vi "LOERN_OnOperate.vi"(0 "XRef":T8, 1 "Point":T6, 2 "State In":T1={"Inputs"=1, "SelectedIndex"=1, "ClassInfo"=[]}) -> (14 "Reply":T4, 15 "Fatal Error Out":T3, 16 "State Out":T1={"Inputs"=1, "SelectedIndex"=1, "ClassInfo"=[]})   [LabVIEW 2016, in "LV Object Event Registration Node.xnode"]
uses:
  LV Object Event Registration Node.xnode
  <vilib>/XNodeSupport/XNodeXNodeRef.ctl
  <vilib>/XNodeSupport/XNodePoint.ctl
  <vilib>/XNodeSupport/XNodeInt.ctl
  LOERN_State.ctl
  LOERN_ClassInfo.ctl
  <vilib>/XNodeSupport/XNodeStringArray.ctl
  <vilib>/XNodeSupport/XNodeString.ctl
  <vilib>/XNodeSupport/XNodeErrorCluster.ctl
  <vilib>/XNodeSupport/NI_XNodeSupport.lvlib
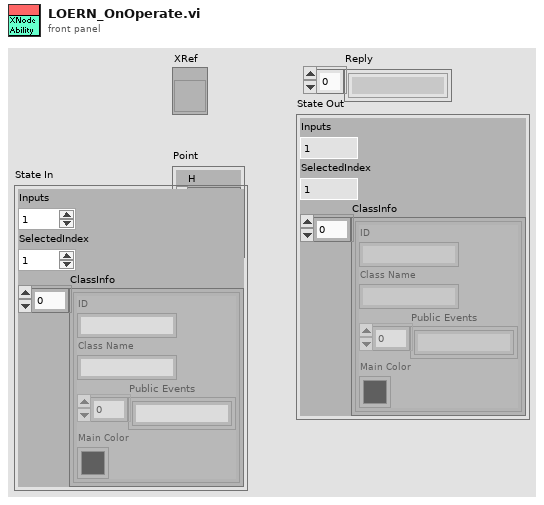
[diagram p1: front panel]
types:
  T1 = typedef "LV Object Event Registration Node.xnode/LOERN_State.ctl" = cluster{"Inputs":u16, "SelectedIndex":i16, "ClassInfo":T2[]}
  T2 = typedef "LV Object Event Registration Node.xnode/LOERN_ClassInfo.ctl" = cluster{"ID":string, "Class Name":string, "Public Events":string[], "Main Color":u32}
  T3 = typedef "NI_XNodeSupport.lvlib/XNodeErrorCluster.ctl" = errorcluster
  T4 = typedef "NI_XNodeSupport.lvlib/XNodeStringArray.ctl" = T5[]
  T5 = typedef "NI_XNodeSupport.lvlib/XNodeString.ctl" = string
  T6 = typedef "NI_XNodeSupport.lvlib/XNodePoint.ctl" = cluster{"H":T7, "V":T7}
  T7 = typedef "NI_XNodeSupport.lvlib/XNodeInt.ctl" = i32
  T8 = typedef "NI_XNodeSupport.lvlib/XNodeXNodeRef.ctl" = refnum<vi>
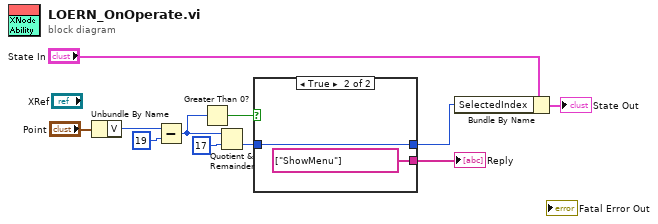
[diagram p0: block diagram]
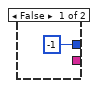
[diagram p2: hidden frame]
diagram:
  n1 = Unbundle By Name("Point") -> ("V"=w10:T7)
  n2 = Subtract(x=w10, y=19) -> (x-y=w7:T7)
  n3 = Greater Than 0?(x=w7) -> (x > 0?=w6:bool)
  n4 = Quotient & Remainder(x=w7, y=17) -> (floor(x/y)=w4:T7)  [unwired: 1 out]
  n5 = case shown="True" w6 {
    tunnel: [_ T4 ["ShowMenu"] ("Reply")] -> w5
    tunnel: w4 -> [_ w13]
    tunnel: [T7 -1 ("V") w13] -> w3
    frame False {
    }
    frame True {
    }
  }
  "Reply" <- w5
  n6 = Bundle By Name(cluster="State In", "SelectedIndex"=w3) -> (→"State Out":T1)
